vi "Swerve Drive.vi"(0 "X":dbl(slide)=0.5 scale=-1.0..1.0, 3 "Y":dbl(slide) scale=1.0..-1.0, 6 "Z":dbl(knob) scale=1.0..-1.0, 10 "Rot. Point Y":dbl, 11 "Auto Controls":bool=TRUE, 13 "Robot-Centric":bool, 16 "Rot. Point X":dbl) -> (20 "Back left Spin Power":dbl=-0.0, 21 "Back Right Spin Power":dbl=-0.0, 22 "Front left Spin Power":dbl=-0.0, 23 "Front Right Spin Power":dbl=-0.0, 24 "Back left Motor Power":dbl=-0.59, 25 "Back Right Motor Power":dbl=0.5, 26 "Front left Motor Power":dbl=0.59, 27 "Front Right Motor Power":dbl=-0.5)   [LabVIEW 2014]
doc: "Main block for a swerve drive. X, Y, and Z are the only inputs that must be wired.\nX and Y are the joystick axes for translational (strafing) movement. Z is the joystick axis for rotation. Rotation point is the point relative to the center of the robot (in inches), around which the robot rotates. This input is optional, leave it blank to always rotate around the center of the robot. If Auto Controls is true, then the inputs will not be squared, and there will be no deadband. If Robot-Centric is true, then the gyro will be ignored, and pushing forward on the joystick will result in a foward movement relative to the robot's direction."
uses:
  Global Variables/Sensor Data (Edited).vi
  Global Variables/Settings.vi
panel:
  out "Front Right PID Tracking":cluster{"Goal Wheel Position":dbl, dbl}(graph)={"Goal Wheel Position"=0.0, -90.17571233858979}
  in  "Robot Length":dbl=22.0
  in  "Robot Width":dbl=37.5
  # "SWERVE DRIVE\nVersion 3.1\n\nCory Lynch\nApple Pi Robotics\nTeam 2067"
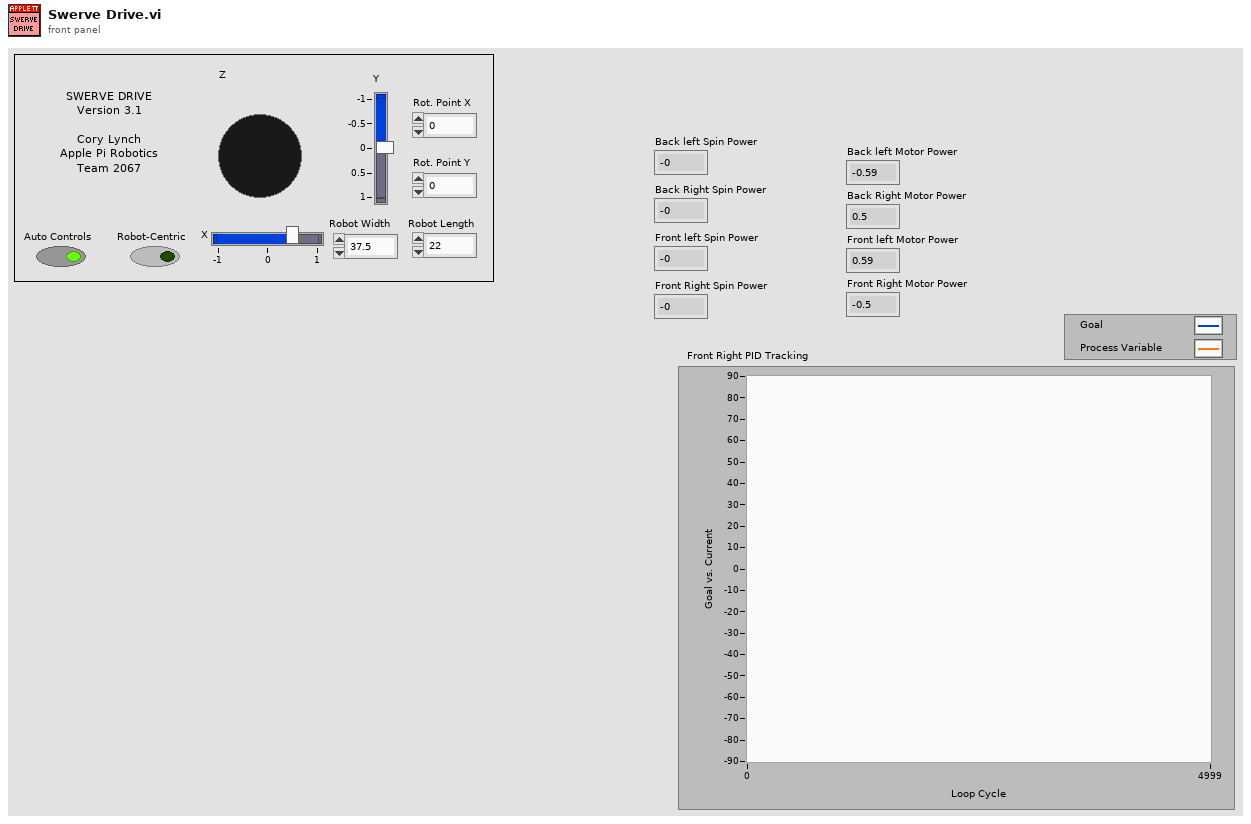
[diagram p1: front panel]
types:
  T1 = enum16{"Back Left", "Back Right", "Front Left", "Front Right"}
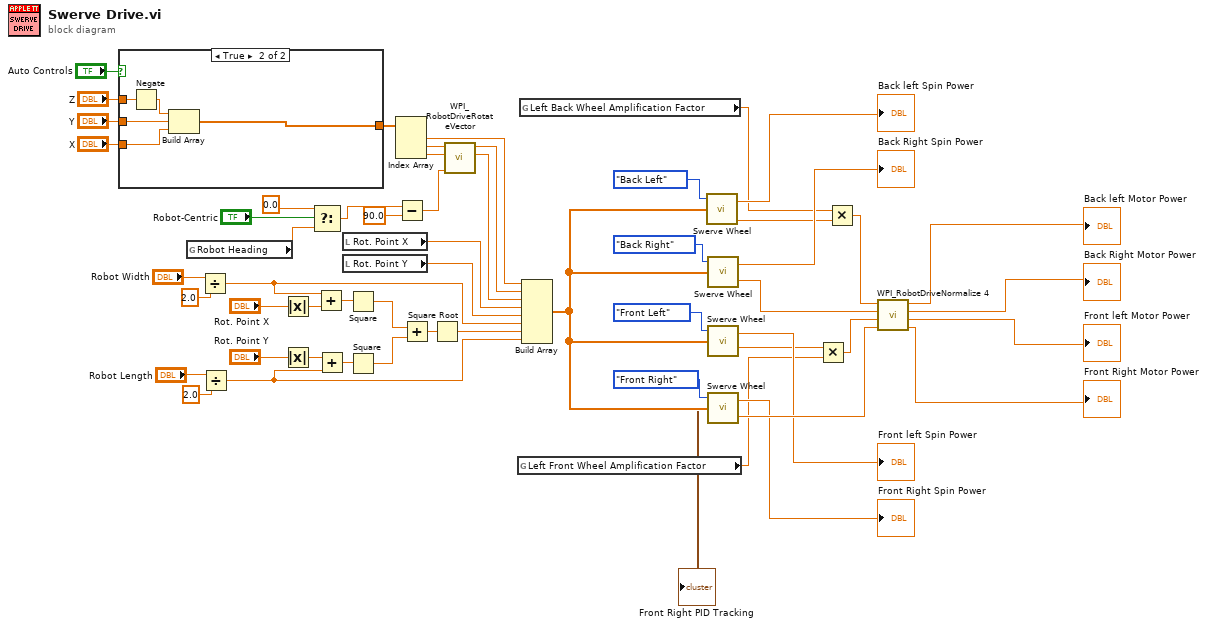
[diagram p0: block diagram]
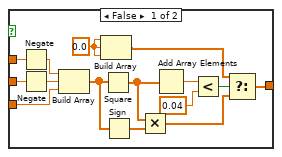
[diagram p2: hidden frame]
diagram:
  n1 = case shown="True" "Auto Controls" {
    tunnel: "Y" -> [w68 w73]
    tunnel: "X" -> [w62 w76]
    tunnel: "Z" -> [w61 w75]
    tunnel: [w58 w72] -> w32
    frame False {
      w66 = 0.0 ("element")
      n2 = Negate(x=w61) -> (-x=w57:dbl)
      n3 = Negate(x=w68) -> (-x=w60:dbl)
      n4 = Build Array(w57, w60, w62) -> (w65:dbl[])
      n5 = Build Array(w66, w66, w66) -> (w67:dbl[])
      n6 = Square(x=w65) -> (x^2=w63:dbl[])
      n7 = Sign(1:w65) -> (0:w64:dbl[])
      n8 = Multiply(x=w63, y=w64) -> (x*y=w59:dbl[])
      n9 = Add Array Elements(numeric array=w63) -> (sum=w71:dbl)
      n10 = Less?(x=w71, y=0.04 ("x")) -> (x < y?=w69:bool)
      n11 = Select(t=w67, s=w69, f=w59) -> (s? t:f=w58:dbl[])
    }
    frame True {
      n12 = Negate(x=w75) -> (-x=w74:dbl)
      n13 = Build Array(w74, w73, w76) -> (w72:dbl[])
    }
  }
  n14 = global read "Sensor Data (Edited).vi" "Robot Heading"() -> (w24:dbl)
  n15 = Divide(x="Robot Width", y=2.0) -> (x/y=w36:dbl)
  n16 = Divide(x="Robot Length", y=2.0) -> (x/y=w34:dbl)
  n17 = Absolute Value(x="Rot. Point X") -> (abs(x)=w54:dbl)
  n18 = Absolute Value(x="Rot. Point Y") -> (abs(x)=w52:dbl)
  n19 = Select(t=0.0, s="Robot-Centric", f=w24) -> (s? t:f=w12:dbl)
  n20 = Add(x=w36, y=w54) -> (x+y=w53:dbl)
  n21 = Add(x=w52, y=w34) -> (x+y=w51:dbl)
  n22 = local read "Rot. Point X"() -> (w38:dbl)
  n23 = local read "Rot. Point Y"() -> (w37:dbl)
  n24 = Square(x=w53) -> (x^2=w49:dbl)
  n25 = Square(x=w51) -> (x^2=w50:dbl)
  n26 = Index Array(array=w32) -> (element #1=w27:dbl, element #2=w33:dbl, element #3=w41:dbl)  [unwired: 3 in]
  n27 = Subtract(x=w12, y=90.0) -> (x-y=w11:dbl)
  n28 = Add(x=w49, y=w50) -> (x+y=w48:dbl)
  n29 = Square Root(x=w48) -> (sqrt(x)=w35:dbl)
  n30 = call <vilib>:"WPI_RobotDriveRotateVector.vi"("Angle"=w11, "X"=w41, "Y"=w33) -> ("X'"=w30:dbl, "Y'"=w26:dbl)  [unwired: 7 out]
  n31 = global read "Settings.vi" "Left Front Wheel Amplification Factor"() -> (w5:dbl)
  n32 = global read "Settings.vi" "Left Back Wheel Amplification Factor"() -> (w2:dbl)
  n33 = Build Array(w27, w26, w30, w38, w37, w36, w35, w34) -> (w31:dbl[])
  n34 = call "Swerve Wheel.vi"("Inputs"=w31, "Wheel"=T1."Back Left") -> ("Speed"=w3:dbl, "Spin Motor Power"=→"Back left Spin Power":dbl)  [unwired: 1 in, 1 out]
  n35 = call "Swerve Wheel.vi"("Inputs"=w31, "Wheel"=T1."Back Right") -> ("Speed"=w19:dbl, "Spin Motor Power"=→"Back Right Spin Power":dbl)  [unwired: 1 in, 1 out]
  n36 = call "Swerve Wheel.vi"("Inputs"=w31, "Wheel"=T1."Front Left") -> ("Speed"=w4:dbl, "Spin Motor Power"=→"Front left Spin Power":dbl)  [unwired: 1 in, 1 out]
  n37 = call "Swerve Wheel.vi"("Inputs"=w31, "Wheel"=T1."Front Right") -> ("Speed"=w56:dbl, "Spin Motor Power"=→"Front Right Spin Power":dbl, "PID Tracking"=→"Front Right PID Tracking":cluster{"Goal Wheel Position":dbl, dbl})  [unwired: 1 in]
  n38 = Multiply(x=w4, y=w5) -> (x*y=w6:dbl)
  n39 = Multiply(x=w2, y=w3) -> (x*y=w7:dbl)
  n40 = call <vilib>:"WPI_RobotDriveNormalize 4.vi"("D"=w56, "C"=w6, "B"=w19, "A"=w7) -> ("D'"=→"Front Right Motor Power":dbl, "C'"=→"Front left Motor Power":dbl, "B'"=→"Back Right Motor Power":dbl, "A'"=→"Back left Motor Power":dbl)
